vi "Emballage_BDD_GVF_bool_Réseau_annule_visualiser.vi"(0 "SetGet":T1=enum."get", 5 "Visualiser IN":bool, 9 "annuler le test car pas d'accès (T) IN":bool, 11 "Error in":errorcluster caption="Error in (no error)") -> (6 "Visualiser OUT":bool, 10 "annuler le test car pas d'accès (T) OUT":bool, 15 "Error out":errorcluster)   [LabVIEW 2020]
uses:
  Modules/FS/60_FS_Controles/60_FS_SetGet.ctl
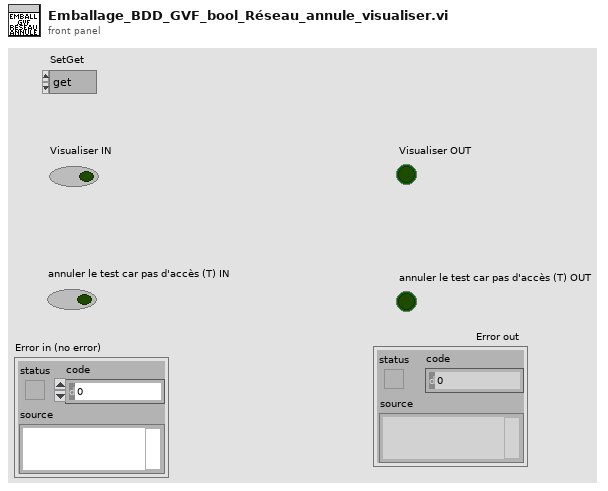
[diagram p1: front panel]
types:
  T1 = typedef "60_FS_SetGet.ctl" = enum16{"set", "get"}
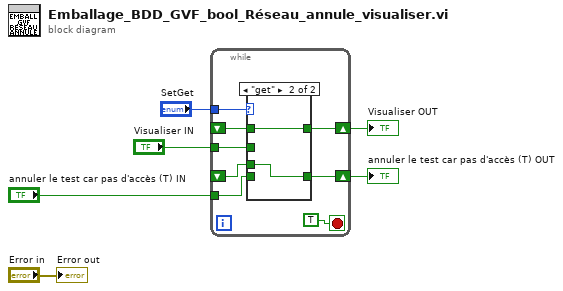
[diagram p0: block diagram]
diagram:
  n1 = while {
    tunnel: "SetGet" -> [w13]
    tunnel: "annuler le test car pas d'accès (T) IN" -> [w11]
    tunnel: "Visualiser IN" -> [w9]
    shift-right: [w10] -> w2
    shift-left: _ -> [w8]
    shift-right: [w12] -> w4
    shift-left: _ -> [w7]
    stop <- TRUE stop-if-true
    n2 = case shown="\"get\"" w13 {
      tunnel: [w16 w17] -> w12
      tunnel: w11 -> [w16 _]
      tunnel: [w15 w18] -> w10
      tunnel: w9 -> [w15 _]
      tunnel: w8 -> [_ w18]
      tunnel: w7 -> [_ w17]
      frame "set", Default {
      }
      frame "get" {
      }
    }
  }
  "Visualiser OUT" <- w2
  "annuler le test car pas d'accès (T) OUT" <- w4
  "Error out" <- "Error in"
